vi "Read Relative Measurement.vi"(0 "VISA resource name":refnum<visa-resource-name>, 11 "error in (no error)":errorcluster) -> (4 "VISA resource name out":refnum<visa-resource-name>, 6 "Relative Measurements":cluster{dbl[], dbl[]}(graph), 15 "error out":errorcluster)   [LabVIEW 2020, in "Keithley 648X Series.lvlib"]
doc: "Initiates the instrument and reads the fresh relative readings."
uses:
  <instrlib>/Keithley 648X Series/Keithley 648X Series.lvlib
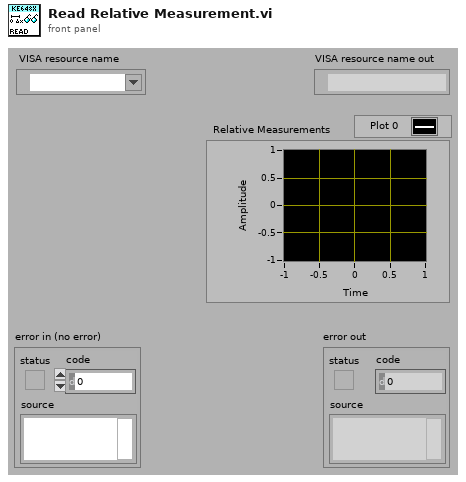
[diagram p1: front panel]
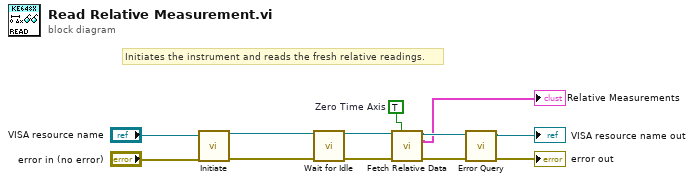
[diagram p0: block diagram]
diagram:
  w1 = TRUE  # Zero Time Axis
  # "Initiates the instrument and reads the fresh relative readings."
  n1 = call <instrlib>:"Initiate.vi"("VISA resource name"="VISA resource name", "error in (no error)"="error in (no error)") -> ("VISA resource name out"=w7:refnum<visa-resource-name>, "error out"=w8:errorcluster)  [unwired: 12 in]
  n2 = call <instrlib>:"Wait for Idle.vi"("VISA resource name"=w7, "error in (no error)"=w8) -> ("VISA resource name out"=w4:refnum<visa-resource-name>, "error out"=w5:errorcluster)  [unwired: 12 in]
  n3 = call <instrlib>:"Fetch Relative Data.vi"("VISA resource name"=w4, "Zero Time Axis (T)"=w1, "error in (no error)"=w5) -> ("VISA resource name out"=w3:refnum<visa-resource-name>, "Relative Data"=→"Relative Measurements":cluster{dbl[], dbl[]}, "error out"=w6:errorcluster)  [unwired: 10 in]
  n4 = call <instrlib>:"Error Query.vi"("error in (no error)"=w6, "VISA resource name"=w3) -> ("error out"=→"error out":errorcluster, "VISA resource name out"=→"VISA resource name out":refnum<visa-resource-name>)  [unwired: 6 in, 2 out]
